vi "WILT Configuration Search SM States.vi"(8 "Error In":errorcluster, 11 "Full Data States":string[](array[string])) -> (0 "Error Out":errorcluster, 3 "SM String":string)   [LabVIEW 2016]
uses:
  <vilib>/Utility/error.llb/whitespace.ctl
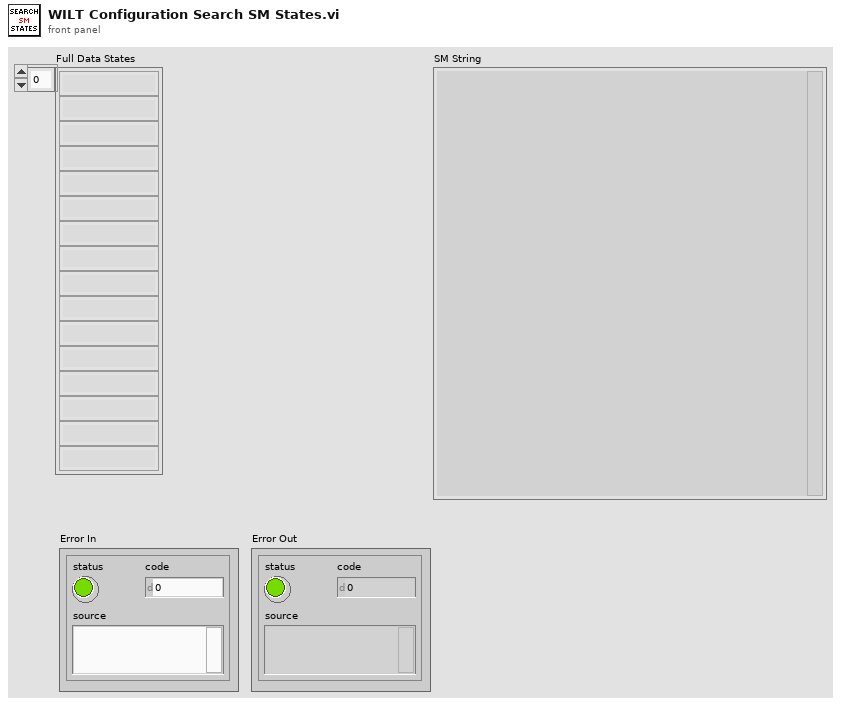
[diagram p1: front panel]
types:
  T1 = typedef "whitespace.ctl" = u16
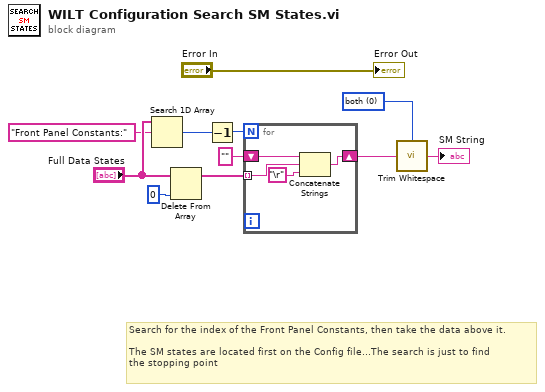
[diagram p0: block diagram]
diagram:
  w6 = T1 0 items=["both", "start of string", "end of string"] ("location (both)")
  # "Search for the index of the Front Panel Constants, then take the data above it.\n\nThe SM states are located first on the Config file...The search is just to find\nthe stopping point"
  n1 = Search 1D Array(1D array="Full Data States", element="Front Panel Constants:") -> (index of element=w10:i32)  [unwired: 1 in]
  n2 = Delete From Array(array="Full Data States", index=0) -> (array with subset deleted=w8:string[])  [unwired: 1 in, 1 out]
  n3 = Decrement(x=w10) -> (x-1=w9:i32)
  n4 = for {
    N: w9 -> [_]
    tunnel: w8 -> [w14] mode=indexing
    shift-right: [w12] -> w4
    shift-left: "" -> [w15]
    n5 = Concatenate Strings(w15, w14, "\r") -> (w12:string)
  }
  n6 = call <vilib>:"Trim Whitespace.vi"("string"=w4, "location (both)"=w6) -> ("trimmed string"=→"SM String":string)
  "Error Out" <- "Error In"
